vi "drive to tape.vi"() -> (1 "y output":dbl, 3 "x output":dbl)   [LabVIEW 2018]
uses:
  Robot Global Data.vi
panel:
  out "Status":dbl
  out "%error":dbl
  out "sees tape":bool
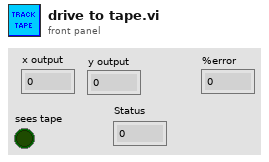
[diagram p1: front panel]
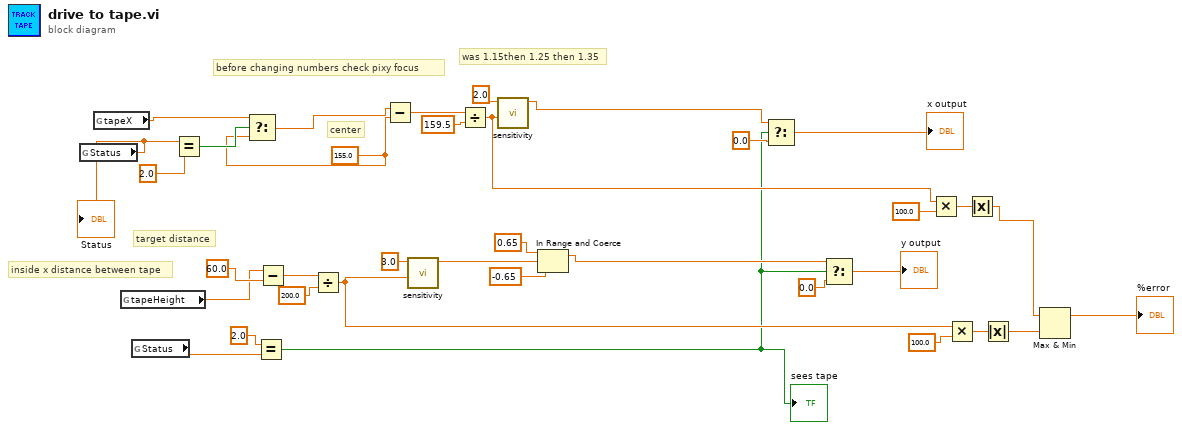
[diagram p0: block diagram]
diagram:
  w2 = 155.0 ("y")
  # "target distance"
  # "was 1.15then 1.25 then 1.35"
  # "center"
  # "inside x distance between tape"
  # "before changing numbers check pixy focus"
  n1 = global read "Robot Global Data.vi" "Status"() -> (w1:dbl)
  "Status" <- w1
  n2 = global read "Robot Global Data.vi" "tapeX"() -> (w4:dbl)
  n3 = global read "Robot Global Data.vi" "tapeHeight"() -> (w7:dbl)
  n4 = global read "Robot Global Data.vi" "Status"() -> (w29:dbl)
  n5 = Equal?(x=w1, y=2.0) -> (x = y?=w6:bool)
  n6 = Select(t=w4, s=w6, f=w2) -> (s? t:f=w5:dbl)
  n7 = Equal?(x=2.0 ("Status"), y=w29) -> (x = y?=w10:bool)
  "sees tape" <- w10
  n8 = Subtract(x=w7, y=60.0) -> (x-y=w28:dbl)
  n9 = Divide(x=w28, y=200.0) -> (x/y=w25:dbl)
  n10 = Subtract(x=w5, y=w2) -> (x-y=w35:dbl)
  n11 = call "sensitivity.vi"("x"=w25, "sensitivity"=3.0) -> ("scaled value"=w14:dbl)  [unwired: 9 in]
  n12 = Divide(x=w35, y=159.5) -> (x/y=w17:dbl)
  n13 = call "sensitivity.vi"("x"=w17, "sensitivity"=2.0) -> ("scaled value"=w31:dbl)  [unwired: 9 in]
  n14 = In Range and Coerce(upper limit=0.65, x=w14, lower limit=-0.65) -> (coerced(x)=w13:dbl)  [unwired: 1 out]
  n15 = Select(t=w31, s=w10, f=0.0) -> (s? t:f=→"x output":dbl)
  n16 = Select(t=w13, s=w10, f=0.0) -> (s? t:f=→"y output":dbl)
  n17 = Multiply(x=w17, y=100.0) -> (x*y=w19:dbl)
  n18 = Multiply(x=w25, y=100.0) -> (x*y=w23:dbl)
  n19 = Absolute Value(x=w19) -> (abs(x)=w18:dbl)
  n20 = Absolute Value(x=w23) -> (abs(x)=w22:dbl)
  n21 = Max & Min(x=w18, y=w22) -> (max(x,y)=→"%error":dbl)  [unwired: 1 out]
